vi "Hote_GetFileWebDAV.vi"(3 "error in":errorcluster caption="entrée d'erreur (pas d'erreur)", 5 "NewValiseFile":path) -> (0 "error out":errorcluster caption="sortie d'erreur", 2 "NewValiseFileOUT":path)   [LabVIEW 2017]
uses:
  <vilib>/WebDAVClient/Simple Get File.vi
  <vilib>/WebDAVClient/NI_WebDAV.lvlib
  <vilib>/WebDAVClient/Simple Get Multiple Files.vi
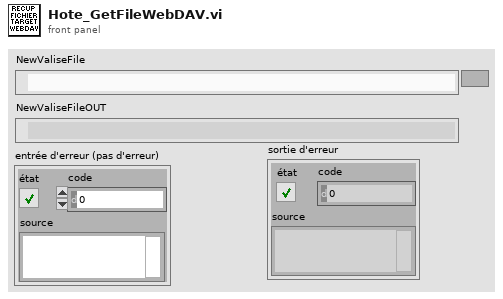
[diagram p1: front panel]
types:
  T1 = cluster{"relative remote file uri":string, "local file path":path}[]
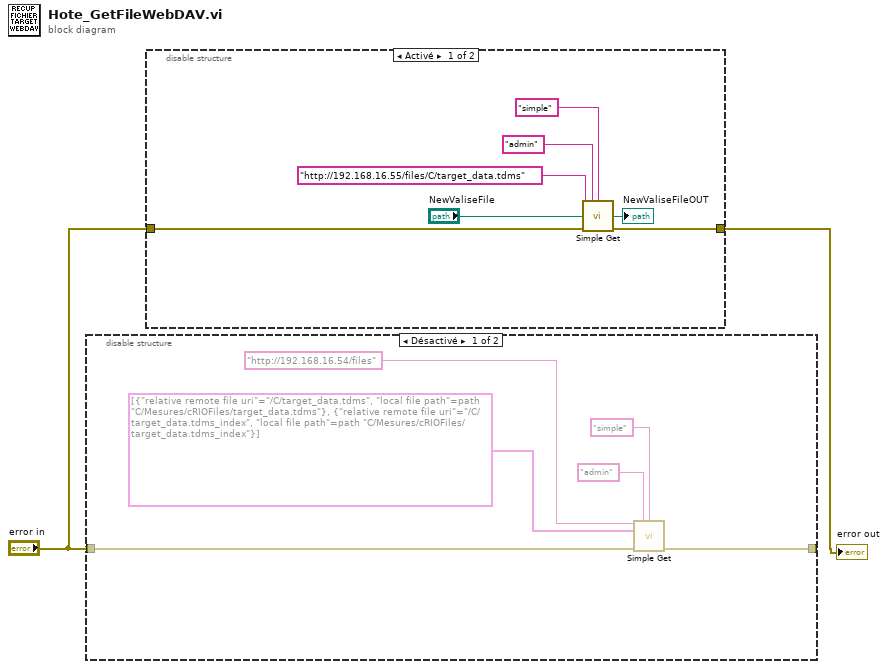
[diagram p0: block diagram]
diagram:
  n1 = disable-structure shown="Désactivé" {
    disable-tunnel: "error in" -> [w4 _]
    disable-tunnel: [w3 _] -> _
    frame Disabled {
      n2 = call-poly <vilib>:"Simple Get.vi"("host uri"="http://192.168.16.54/files", "username"="admin", "password"="simple", "file specifications"=T1 [{"relative remote file uri"="/C/target_data.tdms", "local file path"=path "C:/Mesures/cRIOFiles/target_data.tdms"}, {"relative remote file uri"="/C/target_data.tdms_index", "local file path"=path "C:/Mesures/cRIOFiles/target_data.tdms_index"}], "error in (no error)"=w4) -> ("error out"=w3:errorcluster)  [unwired: 10 in]
    }
    frame Enabled {
    }
  }
  n3 = disable-structure shown="Activé" {
    disable-tunnel: "error in" -> [w10 _]
    disable-tunnel: [w12 _] -> w1
    frame Enabled {
      n4 = call-poly <vilib>:"Simple Get.vi"("remote file uri"="http://192.168.16.55/files/C/target_data.tdms", "username"="admin", "password"="simple", "local file path"="NewValiseFile", "error in (no error)"=w10) -> ("local file path out"=→"NewValiseFileOUT":path, "error out"=w12:errorcluster)  [unwired: 9 in]
    }
    frame Disabled {
    }
  }
  "error out" <- w1
